vi "svx_SC Line Set Scale.vi"(4 "start point":enum16{"center", "top", "bottom"}(ring), 6 "boundary":cluster{"x axis":dbl, "y axis":dbl}, 7 "Selection":enum16{"Autoscale", "X Scale", "Y Scale"}(ring), 8 "Y Min":dbl, 9 "Y Max":dbl, 11 "X Max":dbl) -> (0 "Y Minimum":dbl, 1 "Y Maximum":dbl, 2 "X Minimum":dbl, 3 "X Maximum":dbl)   [LabVIEW 2017, in "SVX SC Line.xctl"]
uses:
  <vilib>/addons/_XControls/Shaft Centerline/SVX SC Line.xctl
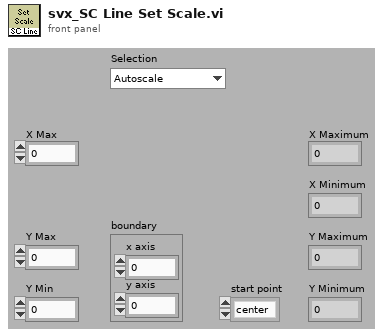
[diagram p1: front panel]
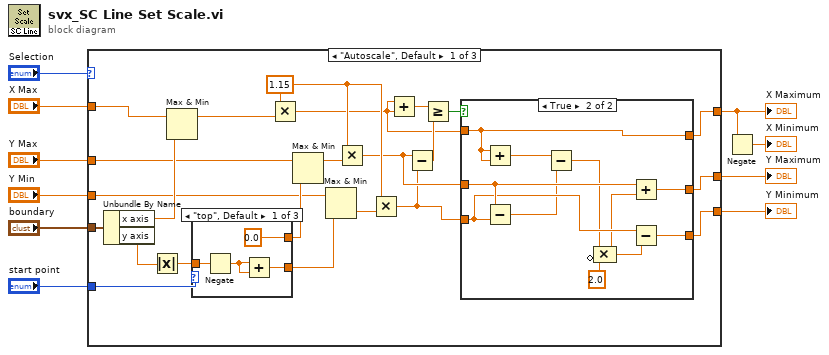
[diagram p0: block diagram]
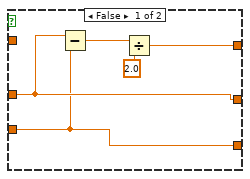
[diagram p2: hidden frame]
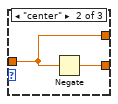
[diagram p3: hidden frame]
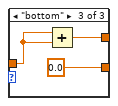
[diagram p4: hidden frame]
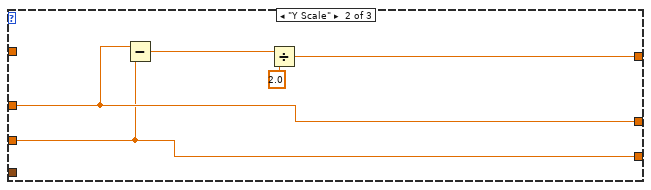
[diagram p5: hidden frame]
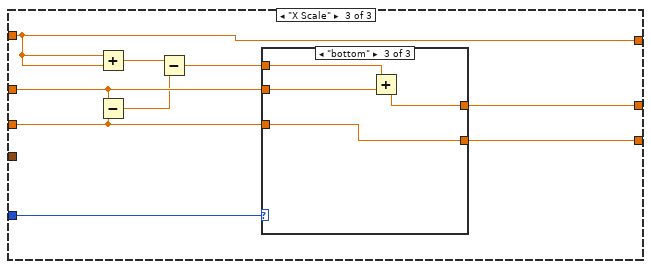
[diagram p6: hidden frame]
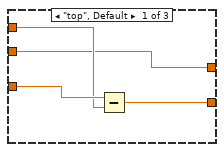
[diagram p7: hidden frame]
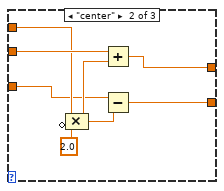
[diagram p8: hidden frame]
diagram:
  n1 = case shown="\"Autoscale\", Default" "Selection" {
    tunnel: "X Max" -> [w32 _ w67]
    tunnel: "Y Max" -> [w24 w60 w71]
    tunnel: "Y Min" -> [w23 w58 w63]
    tunnel: [w13 w62 w67] -> w4
    tunnel: [w12 w60 w70] -> w7
    tunnel: [w11 w58 w69] -> w6
    tunnel: "boundary" -> [w33 _ _]
    tunnel: "start point" -> [w29 _ w64]
    frame "Autoscale", Default {
      w20 = 1.15 ("x")
      n2 = Unbundle By Name(w33) -> ("x axis"=w31:dbl, "y axis"=w28:dbl)
      n3 = Absolute Value(x=w28) -> (abs(x)=w27:dbl)
      n4 = Max & Min(x=w32, y=w31) -> (max(x,y)=w30:dbl)  [unwired: 1 out]
      n5 = case shown="\"top\", Default" w29 {
        tunnel: w27 -> [w50 w53 w57]
        tunnel: [0.0 ("y axis") w53 w56] -> w26
        tunnel: [w51 w54 0.0] -> w25
        frame "top", Default {
          n6 = Negate(x=w50) -> (-x=w49:dbl)
          n7 = Add(x=w49, y=w49) -> (x+y=w51:dbl)
        }
        frame "center" {
          n8 = Negate(x=w53) -> (-x=w54:dbl)
        }
        frame "bottom" {
          n9 = Add(x=w57, y=w57) -> (x+y=w56:dbl)
        }
      }
      n10 = Multiply(x=w20, y=w30) -> (x*y=w16:dbl)
      n11 = Max & Min(x=w24, y=w26) -> (max(x,y)=w22:dbl)  [unwired: 1 out]
      n12 = Max & Min(x=w23, y=w25) -> (min(x,y)=w21:dbl)  [unwired: 1 out]
      n13 = Multiply(x=w20, y=w22) -> (x*y=w15:dbl)
      n14 = Multiply(x=w20, y=w21) -> (x*y=w14:dbl)
      n15 = Add(x=w16, y=w16) -> (x+y=w19:dbl)
      n16 = Subtract(x=w15, y=w14) -> (x-y=w18:dbl)
      n17 = Greater Or Equal?(x=w19, y=w18) -> (x >= y?=w17:bool)
      n18 = case shown="True" w17 {
        tunnel: w16 -> [_ w41]
        tunnel: w15 -> [w36 w48]
        tunnel: w14 -> [w34 w47]
        tunnel: [w38 w41] -> w13
        tunnel: [w36 w46] -> w12
        tunnel: [w34 w45] -> w11
        frame False {
          n19 = Subtract(x=w36, y=w34) -> (x-y=w35:dbl)
          n20 = Divide(x=w35, y=2.0) -> (x/y=w38:dbl)
        }
        frame True {
          n21 = Add(x=w41, y=w41) -> (x+y=w40:dbl)
          n22 = Subtract(x=w48, y=w47) -> (x-y=w39:dbl)
          n23 = Subtract(x=w40, y=w39) -> (x-y=w44:dbl)
          n24 = Compound Arithmetic op=MULTIPLY(w44, invert 2.0 ("y")) -> (w42:dbl)
          n25 = Add(x=w48, y=w42) -> (x+y=w46:dbl)
          n26 = Subtract(x=w47, y=w42) -> (x-y=w45:dbl)
        }
      }
    }
    frame "Y Scale" {
      n27 = Subtract(x=w60, y=w58) -> (x-y=w59:dbl)
      n28 = Divide(x=w59, y=2.0) -> (x/y=w62:dbl)
    }
    frame "X Scale" {
      n29 = Add(x=w67, y=w67) -> (x+y=w66:dbl)
      n30 = Subtract(x=w71, y=w63) -> (x-y=w65:dbl)
      n31 = Subtract(x=w66, y=w65) -> (x-y=w68:dbl)
      n32 = case shown="\"bottom\"" w64 {
        tunnel: w71 -> [w72 w82 w85]
        tunnel: [w72 w81 w83] -> w70
        tunnel: [w75 w80 w86] -> w69
        tunnel: w68 -> [w73 w79 w84]
        tunnel: w63 -> [w74 w76 w86]
        frame "top", Default {
          n33 = Subtract(x=w74, y=w73) -> (x-y=w75:dbl)
        }
        frame "center" {
          n34 = Compound Arithmetic op=MULTIPLY(w79, invert 2.0 ("y")) -> (w77:dbl)
          n35 = Add(x=w82, y=w77) -> (x+y=w81:dbl)
          n36 = Subtract(x=w76, y=w77) -> (x-y=w80:dbl)
        }
        frame "bottom" {
          n37 = Add(x=w84, y=w85) -> (x+y=w83:dbl)
        }
      }
    }
  }
  "X Maximum" <- w4
  "Y Maximum" <- w7
  "Y Minimum" <- w6
  n38 = Negate(x=w4) -> (-x=→"X Minimum":dbl)
